vi "Set Relay.vi"(6 "Relay Numbers":i32[](array[numeric]), 7 "Relay State (On/off)":bool, 8 "error in (no error)":errorcluster, 10 "Address (0)":i32, 11 "VISA resource name":refnum<visa-resource-name>) -> (0 "error out":errorcluster, 3 "VISA resource name out":refnum<visa-resource-name>)   [LabVIEW 2016, in "Environment Chamber.lvlib" / "Climatic Chamber.lvlib"]
doc: "<b>Relay (time signal) setting</B>\n\nEnables or Disables the relay set point in constant mode (No.1)."
uses:
  Climatic Chamber.lvlib
panel:
  out "NACK":bool
  out "Error":bool
  out "ACK":bool
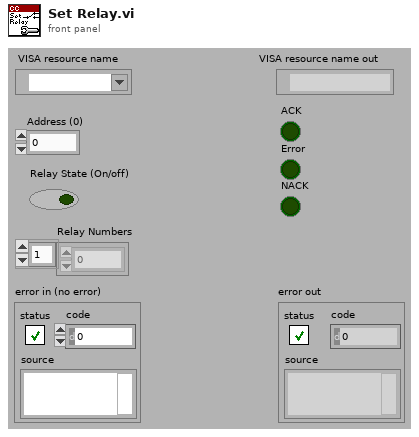
[diagram p1: front panel]
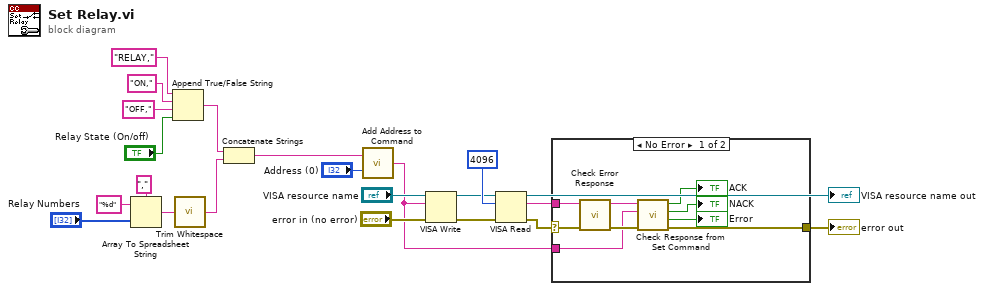
[diagram p0: block diagram]
diagram:
  n1 = Array To Spreadsheet String(delimiter (Tab)=",", array="Relay Numbers", 3:"%d" ("format string")) -> (spreadsheet string=w8:string)
  n2 = Append True/False String(1:"Relay State (On/off)", 2:"OFF,", 3:"ON," ("true string"), 4:"RELAY,") -> (0:w7:string)
  n3 = call <vilib>:"Trim Whitespace.vi"("string"=w8) -> ("trimmed string"=w6:string)  [unwired: 1 in]
  n4 = Concatenate Strings(w7, w6) -> (w5:string)
  n5 = call "Add Address to Command.vi"("Address (0)"="Address (0)", "Command"=w5) -> ("Command OUT"=w12:string)
  n6 = VISA Write(VISA resource name="VISA resource name", write buffer=w12, error in (no error)="error in (no error)") -> (VISA resource name out=w19:refnum<visa-resource-name>, error out=w18:errorcluster)  [unwired: 1 out]
  n7 = VISA Read(VISA resource name=w19, byte count=u32 4096, error in (no error)=w18) -> (VISA resource name out=→"VISA resource name out":refnum<visa-resource-name>, read buffer=w14:string, error out=w15:errorcluster)  [unwired: 1 out]
  n8 = case shown="No Error" w15 {
    selector: w15 -> [w30 w32]
    tunnel: w14 -> [w31 _]
    tunnel: [w26 w32] -> w13
    tunnel: w12 -> [w27 _]
    frame No Error {
      n9 = call "Check Error Response.vi"("error in (no error)"=w30, "read String"=w31) -> ("error out"=w29:errorcluster, "String out"=w28:string)  [unwired: 7 in, 1 out]
      n10 = call "Check Response from Set Command.vi"("error in (no error)"=w29, "Command"=w27, "Response"=w28) -> ("error out"=w26:errorcluster, "Error"=→"Error":bool, "NACK"=→"NACK":bool, "ACK"=→"ACK":bool)  [unwired: 5 in]
    }
    frame Error {
    }
  }
  "error out" <- w13
